vi "Initialize From File.vi"(0 "NIPKG_LV in":refnum<class "NIPKG_LV.lvclass">) -> (4 "NIPKG_LV out":refnum<class "NIPKG_LV.lvclass">)   [LabVIEW 2017, in "CL_G3_VIComponentBuilder.lvlib" / "NIPKG_LV.lvclass"]
doc: "Initializes the class from the configuration file."
uses:
  NIPKG_LV.lvclass
  C:/builds/Component BuilderBT/SrcDist/Exports/Exports/Export.lvclass
  Exports/Export.lvclass/Export.ctl
  NIPKG_LV.lvclass/NIPKG_LV.ctl
  Exports/Accessors/Read Export Config File.vi
  Accessors/Write Build Machine Feed Folderpath.vi
  Exports/Accessors/Write Export Operation Errors.vi
  Exports/Accessors/Read Export Operation Errors.vi
  NI Build Specification_LV/NI Build Specification_LV.lvclass
  <vilib>/Utility/config.llb/NI_LVConfig.lvlib
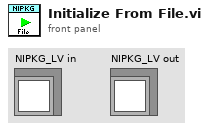
[diagram p1: front panel]
types:
  T1 = typedef "NI_LVConfig.lvlib/Config Data RefNum.ctl" = refnum<k1>
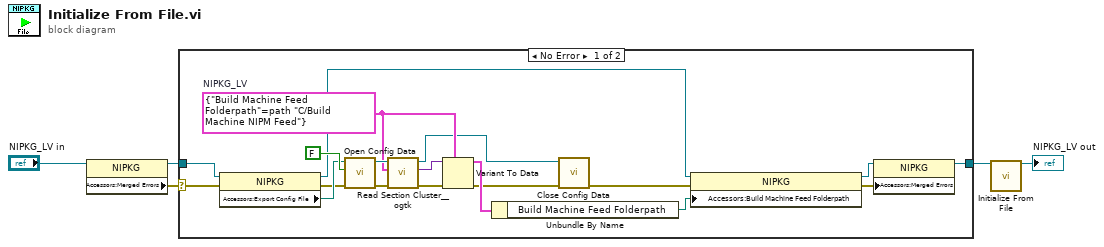
[diagram p0: block diagram]
diagram:
  n1 = property class="NIPKG"(reference="NIPKG_LV in") -> (reference out=w1:refnum<class "NIPKG_LV.lvclass">, "Accessors:Merged Errors"=w2:errorcluster)  [unwired: 1 in, 1 out]
  n2 = case shown="No Error" w2 {
    selector: w2 -> [w6 _]
    tunnel: [w10 w25] -> w4
    tunnel: w1 -> [w24 w25]
    frame No Error {
      w20 = cluster{"Build Machine Feed Folderpath":path} {"Build Machine Feed Folderpath"=path "C:/Build Machine NIPM Feed"}  # NIPKG_LV
      n3 = property class="NIPKG"(reference=w24, error in=w6) -> (reference out=w8:refnum<class "NIPKG_LV.lvclass">, error out=w15:errorcluster, "Accessors:Export Config File"=w16:path)
      n4 = call <vilib>:"Open Config Data.vi"("error in (no error)"=w15, "create file if necessary (T)"=FALSE, "configuration file path"=w16) -> ("error out"=w18:errorcluster, "refnum"=w22:T1)  [unwired: 6 in, 1 out]
      n5 = call <userlib>:"Read Section Cluster__ogtk.vi"("error in (no error)"=w18, "Section Formatted Cluster Type"=w20, "refnum"=w22) -> ("error out"=w17:errorcluster, "Section Formatted Cluster"=w21:variant, "dup refnum"=w13:T1)  [unwired: 4 in, 2 out]
      n6 = Variant To Data(error in=w17, type=w20, Variant=w21) -> (data=w19:cluster{"Build Machine Feed Folderpath":path}, error out=w12:errorcluster)
      n7 = Unbundle By Name(w19) -> ("Build Machine Feed Folderpath"=w14:path)
      n8 = call <vilib>:"Close Config Data.vi"("error in (no error)"=w12, "refnum"=w13) -> ("error out"=w7:errorcluster)  [unwired: 8 in, 1 out]
      n9 = property class="NIPKG"(reference=w8, error in=w7, "Accessors:Build Machine Feed Folderpath"=w14) -> (reference out=w11:refnum<class "NIPKG_LV.lvclass">, error out=w9:errorcluster)
      n10 = property class="NIPKG"(reference=w11, "Accessors:Merged Errors"=w9) -> (reference out=w10:refnum<class "NIPKG_LV.lvclass">)  [unwired: 1 in, 1 out]
    }
    frame Error {
    }
  }
  n11 = call-parent "Initialize From File.vi"("NI Build Specification_LV in"=w4) -> ("NI Build Specification_LV out"=→"NIPKG_LV out":refnum<class "NIPKG_LV.lvclass">)  [unwired: 14 in]
